vi "Entry to String.vi"(10 "error in (no error)":errorcluster, 11 "Entry":T2) -> (2 "error out":errorcluster, 3 "String Entry":T1)   [LabVIEW 2020, in "Tester.lvlib" / "Results.lvclass"]
uses:
  Results.lvclass
  Entry.ctl
  Result.ctl
  String Entry.ctl
  <vilib>/Utility/error.llb/Error Cluster From Error Code.vi
  <vilib>/ErrorRing/Error Ring.xnode
  <vilib>/Utility/Data Type/NI_Data Type.lvlib
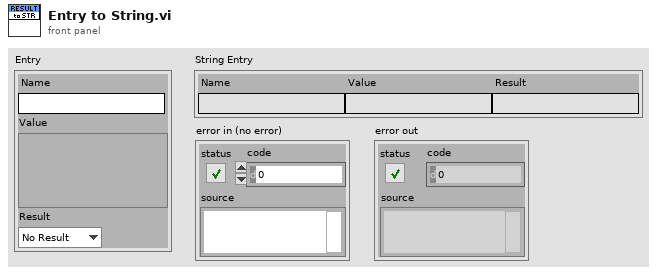
[diagram p1: front panel]
types:
  T1 = typedef "Tester.lvlib/Results.lvclass/String Entry.ctl" = cluster{"Name":string, "Value":string, "Result":string}
  T2 = typedef "Tester.lvlib/Results.lvclass/Entry.ctl" = cluster{"Name":string, "Value":variant, "Result":T3}
  T3 = typedef "Tester.lvlib/Results.lvclass/Result.ctl" = enum16{"No Result", "Pass", "Fail", "Error", "Abort"}
  T4 = typedef "NI_Data Type.lvlib/Data Type.ctl" = enum8{"Invalid Type", "Void", "I8", "I16", "I32", "I64", "U8", "U16", "U32", "U64", "Single Float", "Double Float", "Extended Float", "Single Complex", "Double Complex", "Extended Complex", "Enum U8", "Enum U16", "Enum U32", "Enum U64", "Single Float With Unit", "Double Float With Unit", "Extended Float With Unit", "Single Complex with Unit", "Double Complex with Unit", "Extended Complex with Unit", "Boolean", "String", "Path", "Picture", "Tag", "Array", "Cluster", "Variant", "LV Variant", "Waveform", "Timestamp", "Digital Waveform", "Digital Data", "ExpressData", "Refnum", "External Data", "VI", "Poly VI", "LabVIEW Class Instance", "Fixed Point", "Set Collection", "Map Collection"}
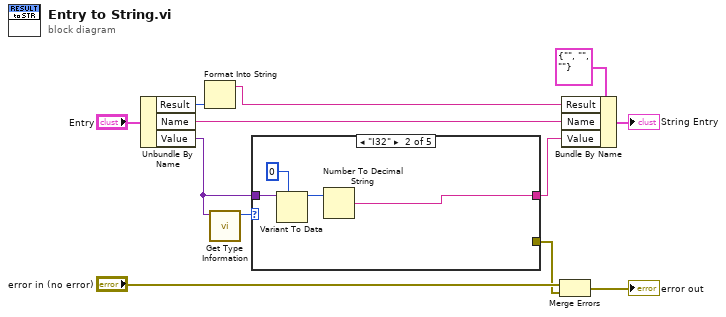
[diagram p0: block diagram]
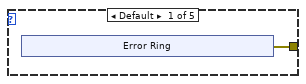
[diagram p2: hidden frame]
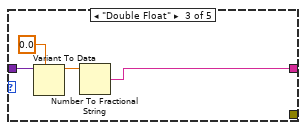
[diagram p3: hidden frame]
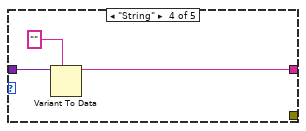
[diagram p4: hidden frame]
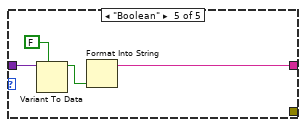
[diagram p5: hidden frame]
diagram:
  n1 = Unbundle By Name("Entry") -> ("Result"=w11:T3, "Name"=w9:string, "Value"=w2:variant)
  n2 = Format Into String(w11) -> (resulting string=w8:string)  [unwired: 3 in, 1 out]
  n3 = call <vilib>:"Get Type Information.vi"("variant"=w2) -> ("type"=w7:T4)  [unwired: 6 in, 4 out]
  n4 = case shown="\"I32\"" w7 {
    tunnel: [w13 _ _ _ _] -> w5
    tunnel: w2 -> [_ w21 w25 w28 w32]
    tunnel: [_ w18 w22 w26 w30] -> w1
    frame Default {
      n5 = xnode "Error Ring"() -> ("error out"=w13:errorcluster)
    }
    frame "I32" {
      n6 = Variant To Data(type=0, Variant=w21) -> (data=w19:i32)  [unwired: 1 in, 1 out]
      n7 = Number To Decimal String(number=w19) -> (decimal integer string=w18:string)  [unwired: 1 in]
    }
    frame "Double Float" {
      n8 = Variant To Data(type=0.0, Variant=w25) -> (data=w23:dbl)  [unwired: 1 in, 1 out]
      n9 = Number To Fractional String(number=w23) -> (F-format string=w22:string)  [unwired: 3 in]
    }
    frame "String" {
      n10 = Variant To Data(type="", Variant=w28) -> (data=w26:string)  [unwired: 1 in, 1 out]
    }
    frame "Boolean" {
      n11 = Variant To Data(type=FALSE, Variant=w32) -> (data=w29:bool)  [unwired: 1 in, 1 out]
      n12 = Format Into String(w29) -> (resulting string=w30:string)  [unwired: 3 in, 1 out]
    }
  }
  n13 = Merge Errors("error in (no error)", w5) -> (→"error out":errorcluster)
  n14 = Bundle By Name(cluster=T1 {"Name"="", "Value"="", "Result"=""} ("String Entry"), "Result"=w8, "Name"=w9, "Value"=w1) -> (→"String Entry":T1)
